vi "KBinsDiscretizer.vi"(8 "error in (no error)":errorcluster caption="entrée d'erreur (pas d'erreur)", 11 "KBinsDiscretizer":T1={"n_bins"=[5], "encode"="onehot", "strategy"="quantile"}) -> (0 "error out":errorcluster, 3 "KBinsDiscretizer.lvclass":refnum<class "KBinsDiscretizer.lvclass">)   [LabVIEW 2020]
doc: "Bin continuous data into intervals.\n\nParameters : \n\n- n_bins : int or array-like, shape (n_features,) (default=5)\nThe number of bins to produce. Raises ValueError if n_bins < 2.\n\n- encode : {‘onehot’, ‘onehot-dense’, ‘ordinal’}, (default=’onehot’)\nMethod used to encode the transformed result.\n\nonehot\nEncode the transformed result with one-hot encoding and return a sparse matrix. Ignored features are always stacked to the right.\n\nonehot-dense\nEncode the transformed result with one-hot encoding and return a dense array. Ignored features are always stacked to the right.\n\nordinal\nReturn the bin identifier encoded as an integer value.\n\n- strategy : {‘uniform’, ‘quantile’, ‘kmeans’}, (default=’quantile’)\nStrategy used to define the widths of the bins.\n\nuniform\nAll bins in each feature have identical widths.\n\nquantile\nAll bins in each feature have the same number of points.\n\nkmeans\nValues in each bin have the same nearest center of a 1D k-means cluster.\n\n\n\nMethods : \n\n\n- Fit : Fit the estimator.\n\nParameters : X : numeric array-like, shape (n_samples, n_features)\n Data to be discretized.\n y : None\n Ignored. \n\n- Fit Transform : Fit to data, then transform it. Fits transformer to X and y with optional parameters fit_params and returns a transformed version of X.\n\nParameters : X : {array-like, sparse matrix, dataframe} of shape (n_samples, n_features)\n y : ndarray of shape (n_samples,), default=None\n Target values.\n\nReturns : X_new : ndarray array of shape (n_samples, n_features_new)\n Transformed array.\n\n\n- Transform : Discretize the data.\n\nParameters : X : numeric array-like, shape (n_samples, n_features)\n Data to be discretized.\n\nReturns : Xt : numeric array-like or sparse matrix\n Data in the binned space."
uses:
  KBinsDiscretizer.lvclass
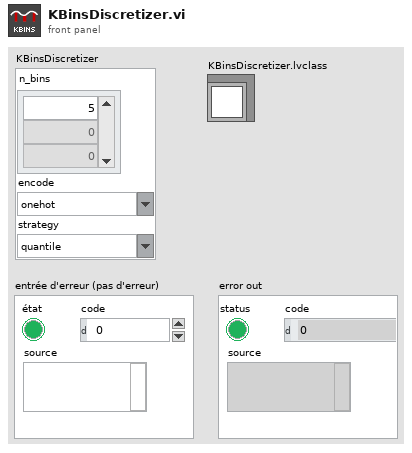
[diagram p1: front panel]
types:
  T1 = cluster{"n_bins":i32[], "encode":string, "strategy":string}
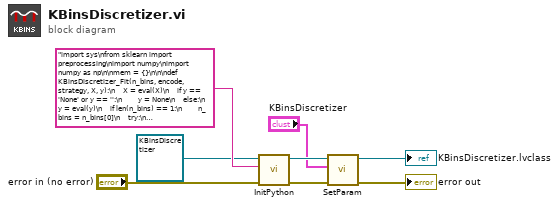
[diagram p0: block diagram]
diagram:
  n1 = call-dynamic "InitPython.vi"("error in (no error)"="error in (no error)", "Python Instruction"="import sys\nfrom sklearn import preprocessing\nimport numpy\nimport numpy as np\n\nmem = {}\n\n\ndef KBinsDiscretizer_Fit(n_bins, encode, strategy, X, y):\n    X = eval(X)\n    if y == 'None' or y == '':\n        y = None\n    else:\n        y = eval(y)\n    if len(n_bins) == 1:\n        n_bins = n_bins[0]\n    try:\n        KBinsDiscretizer= preprocessing.KBinsDiscretizer(n_bins, encode, strategy).fit(X, y)\n        mem['FitKBinsDiscretizer'] = KBinsDiscretizer\n        return str('OK')\n    except:\n        erreur = sys.exc_info()\n        typerr = u\"%s\" % (erreur[0])\n        typerr = typerr[typerr.find(\"'\")+1:typerr.rfind(\"'\")]\n        msgerr = u\"%s\" % (erreur[1])\n        message = str('/!\\\\ {0} : {1}'. format(typerr,msgerr))\n        return message \n    \ndef KBinsDiscretizer_FitTransform(n_bins, encode, strategy, X, y):\n    X = eval(X)\n    if y == 'None' or y == '':\n        y = None\n    else:\n        y = eval(y)\n    if len(n_bins) == 1:\n        n_bins = n_bins[0]\n    try:\n        \n        KBinsDiscretizer = preprocessing.KBinsDiscretizer(n_bins, encode, strategy).fit_transform(X, y)\n        dtype = type(KBinsDiscretizer)\n        if dtype == numpy.ndarray:\n            KBinsDiscretizer = KBinsDiscretizer.tolist()\n            return str(KBinsDiscretizer) \n        else:\n            Mat = KBinsDiscretizer.tocoo()\n            return str(list(zip(Mat.row, Mat.col, Mat.data)))\n    except:\n        erreur = sys.exc_info()\n        typerr = u\"%s\" % (erreur[0])\n        typerr = typerr[typerr.find(\"'\")+1:typerr.rfind(\"'\")]\n        msgerr = u\"%s\" % (erreur[1])\n        message = str('/!\\\\ {0} : {1}'. format(typerr,msgerr))\n        return message \n\ndef KBinsDiscretizer_Transform(n_bins, encode, strategy, X, y):\n    X = eval(X)\n    if y == 'None' or y == '':\n        y = None\n    else:\n        y = eval(y)\n    if len(n_bins) == 1:\n        n_bins = n_bins[0]\n    try:\n        KBinsDiscretizer= mem['FitKBinsDiscretizer'].transform(X)\n        dtype = type(KBinsDiscretizer)\n        if dtype == numpy.ndarray:\n            KBinsDiscretizer = KBinsDiscretizer.tolist()\n            return str(KBinsDiscretizer) \n        else:\n            Mat = KBinsDiscretizer.tocoo()\n            return str(list(zip(Mat.row, Mat.col, Mat.data)))\n    except:\n        erreur = sys.exc_info()\n        typerr = u\"%s\" % (erreur[0])\n        typerr = typerr[typerr.find(\"'\")+1:typerr.rfind(\"'\")]\n        msgerr = u\"%s\" % (erreur[1])\n        message = str('/!\\\\ {0} : {1}'. format(typerr,msgerr))\n        return message ", "Scikit-learn en entrée"=refnum<class "KBinsDiscretizer.lvclass"> refnum ("KBinsDiscretizer.lvclass")) -> ("error out"=w3:errorcluster, "Scikit-learn en sortie"=w5:refnum<class "KBinsDiscretizer.lvclass">)  [unwired: 7 in]
  n2 = call-dynamic "SetParam.vi"("error in (no error)"=w3, "KBinsDiscretizer"="KBinsDiscretizer", "KBinsDiscretizer.lvclass"=w5) -> ("error out"=→"error out":errorcluster, "KBinsDiscretizer.lvclass"=→"KBinsDiscretizer.lvclass":refnum<class "KBinsDiscretizer.lvclass">)  [unwired: 7 in]
